vi "MS Operation Thorlabs.vi"(4 "Calib Params?":bool, 6 "OCT Z PID Gains":cluster{"Kp":dbl, "Kd":dbl, "Ki":dbl}={"Kp"=0.0003, "Kd"=0.0001, "Ki"=0.01}, 8 "error in":errorcluster, 9 "OCT Prev Posit":dbl, 11 "FPGA VI Reference In":refnum<k20>) -> (0 "error out":errorcluster, 1 "OCT Last Posit":dbl, 3 "FPGA VI Reference Out":refnum<k20>)   [LabVIEW 2016]
uses:
  <vilib>/Platform/TimedLoop/XDataNode/timing_clust.ctl
  <vilib>/Platform/TimedLoop/XDataNode/nitl_modes.ctl
  <vilib>/Platform/TimedLoop/XDataNode/wakeup.ctl
  Subsystems/Global Variables.vi
  <vilib>/Utility/error.llb/Error Cluster From Error Code.vi
  <vilib>/rvi/errors/niLvFpgaAdjustHostInterfaceError.vi
  <vilib>/platform/TimedLoop/XDataNode/XDataNode.xnode
  <vilib>/rvi/interface/nirviReadWriteControl/nirviReadWriteControl.xnode
  FPGA Bitfiles/PhantomControlPI_FPGATarget_QuadCtr2_E2412E44.lvbitx
  IRISS_FPGA_IO.vi
  <vilib>/Platform/TimedLoop/XDataNode/XDNodeRunTimeDep.lvlib
  Library/KevinLibraryAll/labview/KevLib01.lvlib
  NiFpgaLv.dll
panel:
  out "x+y 2":dbl[](array[numeric])
  out "x+y":dbl[](array[numeric])
  out "Hydration On/Off":bool
  out "vac cmd":dbl
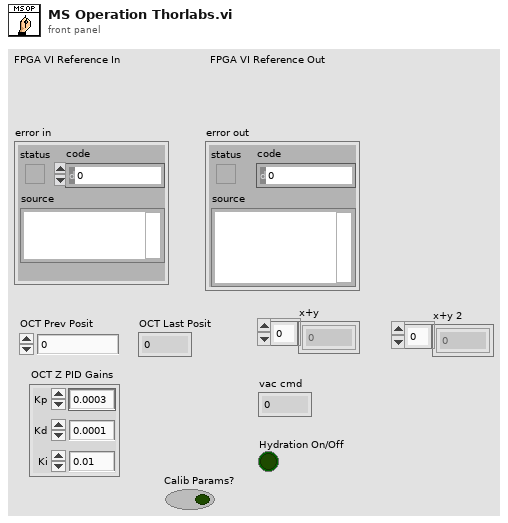
[diagram p1: front panel]
types:
  T1 = typedef "XDNodeRunTimeDep.lvlib/timing_clust.ctl" = cluster{"Expected End [f-1]":u64, "Actual End [f-1]":u64, "Finished Late? [f-1]":bool, "Expected End [i-1]":u64, "Actual End [i-1]":u64, "Finished Late? [i-1]":bool, "Expected Start [i]":u64, "Actual Start [i]":u64, "Expected Start [f]":u64, "Actual Start [f]":u64, "Source Name":string, "Structure Name":string, "Period":i64, "Deadline":i64, "Offset":i64, "Start":i64, "Priority":i32, "Timeout":i32, "Mode":T2, "Wakeup Reason":T3, "Error":errorcluster, "Source Type":string, "Secondary Source Type":string, "Global End Time":u64, "Global Start Time":u64, "Frame Duration":u64, "Iteration Duration":u64, "Assigned CPU":i32, "I/O Scan Engine Mode":u32}
  T2 = typedef "XDNodeRunTimeDep.lvlib/nitl_modes.ctl" = enum32{"No Change", "Process missed periods, maintain original phase", "Discard missed periods, maintain original phase", "Process missed periods, ignore original phase", "Discard missed periods, ignore original phase"}
  T3 = typedef "XDNodeRunTimeDep.lvlib/wakeup.ctl" = enum32{"Normal", "Aborted", "Asynchronous wakeup", "Timing source error", "Timed loop error", "Timeout"}
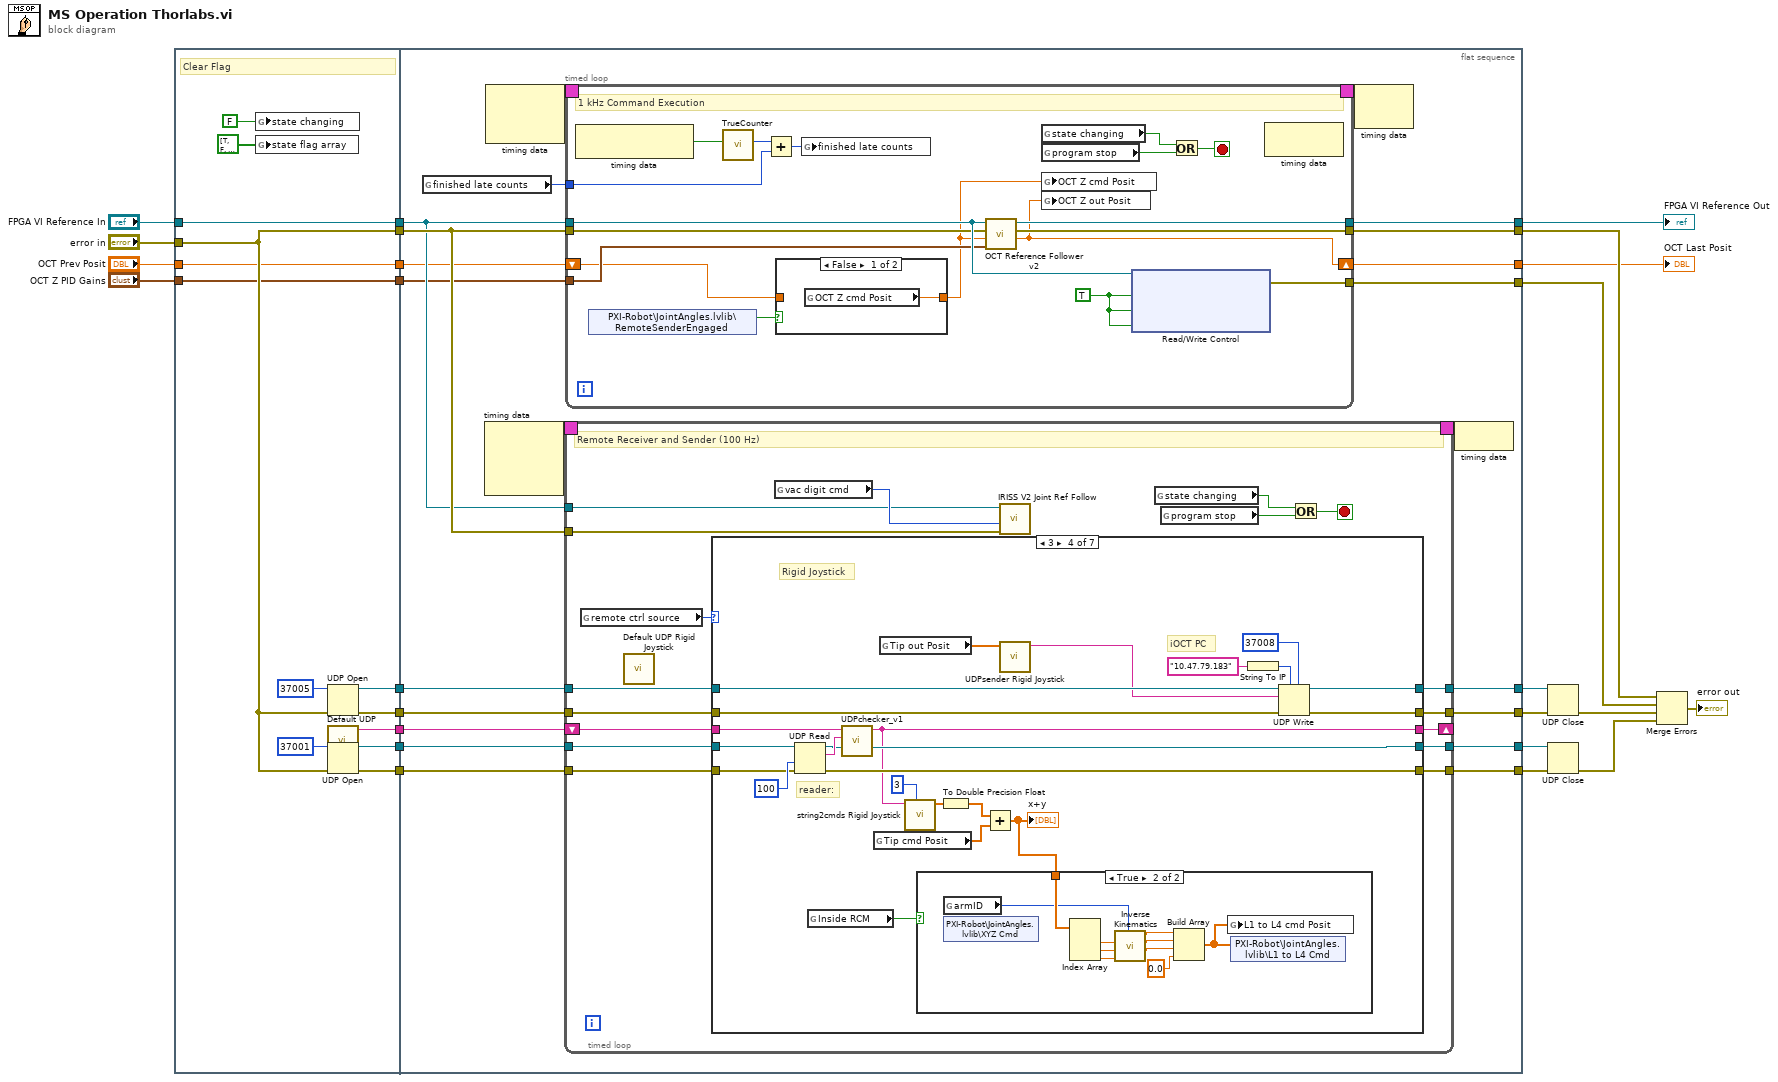
[diagram p0: block diagram]
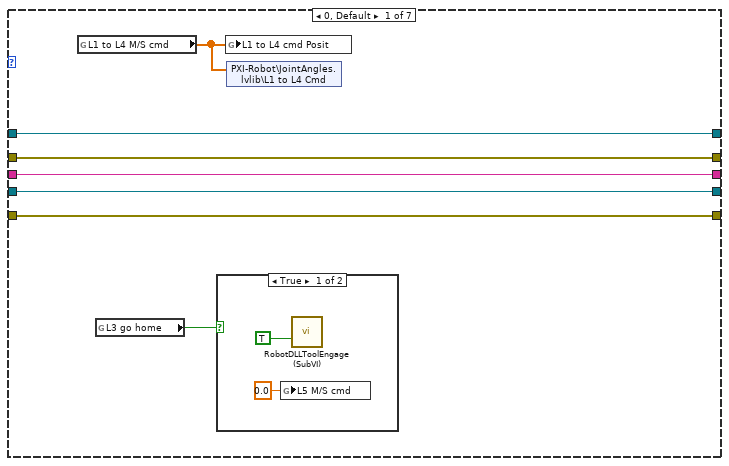
[diagram p2: hidden frame]
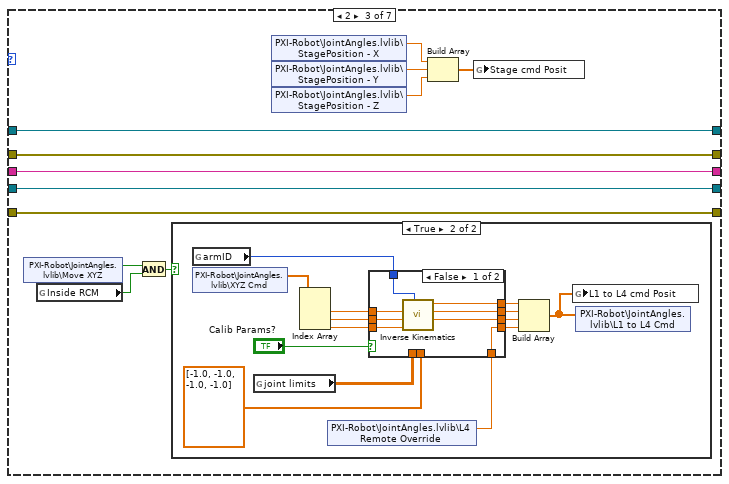
[diagram p5: hidden frame]
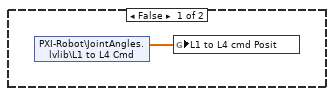
[diagram p6: hidden frame]
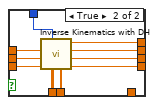
[diagram p7: hidden frame]
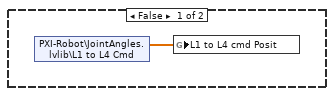
[diagram p8: hidden frame]
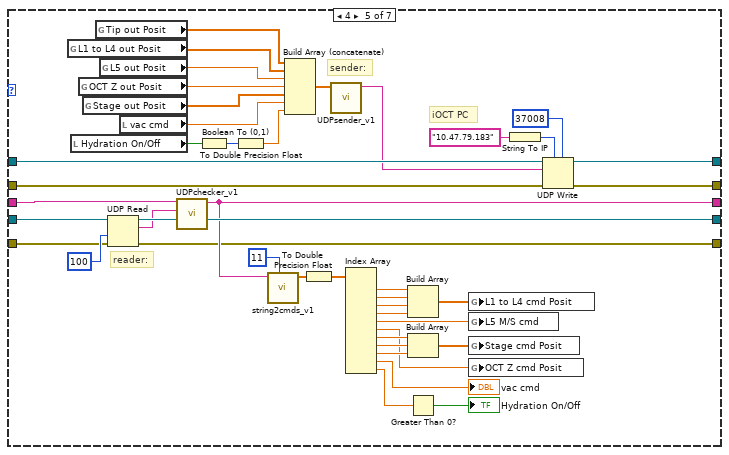
[diagram p9: hidden frame]
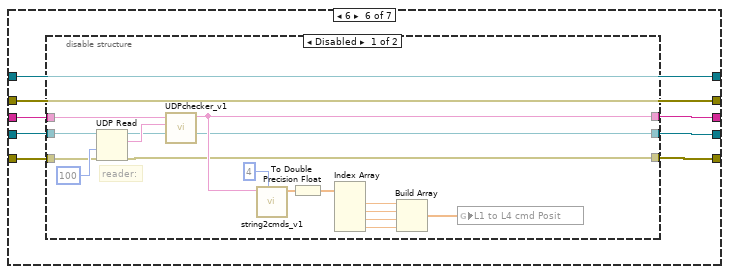
[diagram p10: hidden frame]
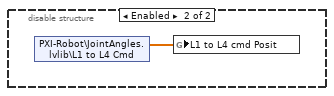
[diagram p11: hidden frame]
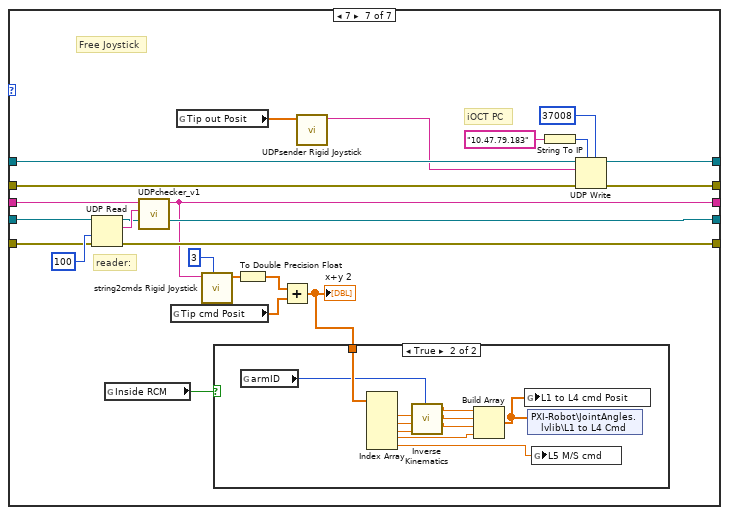
[diagram p12: hidden frame]
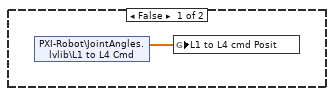
[diagram p13: hidden frame]
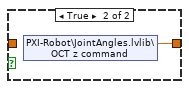
[diagram p14: hidden frame]
diagram:
  n1 = flat-sequence {
    tunnel: [w35] -> w24
    tunnel: "FPGA VI Reference In" -> [w35]
    tunnel: [w27] -> w22
    tunnel: "error in" -> [w27]
    tunnel: [w28] -> w20
    tunnel: [w32] -> w18
    tunnel: [w31] -> w17
    tunnel: [w30] -> w16
    tunnel: [w29] -> w15
    tunnel: [w26] -> w5
    tunnel: "OCT Prev Posit" -> [w26]
    tunnel: [w25] -> w3
    tunnel: "OCT Z PID Gains" -> [w25]
    tunnel: w24 -> [w41]
    tunnel: w22 -> [w42]
    tunnel: [w57] -> w6
    tunnel: [w56] -> w7
    tunnel: [w54] -> w21
    tunnel: w20 -> [w47]
    tunnel: w18 -> [w51]
    tunnel: w17 -> [w50]
    tunnel: w16 -> [w49]
    tunnel: w15 -> [w48]
    tunnel: [w46] -> w12
    tunnel: [w45] -> w11
    tunnel: [w44] -> w10
    tunnel: [w43] -> w9
    tunnel: w5 -> [w40]
    tunnel: w3 -> [w39]
    tunnel: [w38] -> w1
    frame #0 {
      # "Clear Flag"
      n2 = global write "Global Variables.vi" "state changing"(FALSE ("state changing")) -> ()
      n3 = global write "Global Variables.vi" "state flag array"(bool[] [TRUE, FALSE, FALSE, FALSE, FALSE, FALSE, FALSE, FALSE, FALSE, FALSE] ("state flag array")) -> ()
      n4 = UDP Open(8:w27, 11:u16 37005 ("port")) -> (port=w31:refnum<k16>, 0:w32:errorcluster)  [unwired: 3 in, 1 out]
      n5 = call "Default UDP.vi"() -> ("String"=w28:string)  [unwired: 11 in]
      n6 = UDP Open(8:w27, 11:u16 37001 ("port")) -> (port=w30:refnum<k16>, 0:w29:errorcluster)  [unwired: 3 in, 1 out]
    }
    frame #1 {
      n7 = global read "Global Variables.vi" "finished late counts"() -> (w55:u16)
      n8 = node-c288() -> (w53:T1)  [unwired: 3 in]
      n9 = node-c288() -> (w59:T1)  [unwired: 2 in]
      n10 = timed-loop {
        timing: w53 -> [_]
        timing-out: [_] -> w52
        tunnel: w49 -> [w76]
        tunnel: [w75] -> w44
        shift-right: [w73] -> _
        shift-left: w47 -> [w74]
        tunnel: w50 -> [w72]
        tunnel: w51 -> [w71]
        tunnel: [w70] -> w46
        tunnel: [w69] -> w45
        tunnel: w48 -> [w68]
        tunnel: [w67] -> w43
        tunnel: w41 -> [w61]
        tunnel: w42 -> [w60]
        stop <- w64 stop-if-true
        # "Remote Receiver and Sender (100 Hz)"
        n11 = global read "Global Variables.vi" "remote ctrl source"() -> (w63:u16)
        n12 = call "Default UDP Rigid Joystick.vi"() -> ()  [unwired: 11 in, 1 out]
        n13 = case shown="3" w63 {
          tunnel: w76 -> [w80 w87 w99 w156 w211 w217 w258]
          tunnel: [w80 w87 w99 w152 w210 w218 w254] -> w75
          tunnel: w74 -> [w81 w88 w100 w150 w170 w220 w252]
          tunnel: [w81 w88 w100 w149 w197 w219 w251] -> w73
          tunnel: w72 -> [w83 w90 w102 w143 w195 w213 w245]
          tunnel: w71 -> [w82 w89 w101 w141 w194 w214 w243]
          tunnel: [w83 w90 w102 w142 w190 w213 w244] -> w70
          tunnel: [w82 w89 w101 w140 w189 w214 w242] -> w69
          tunnel: w68 -> [w79 w86 w98 w155 w188 w215 w257]
          tunnel: [w79 w86 w98 w151 w187 w216 w253] -> w67
          frame 0, Default {
            n14 = global read "Global Variables.vi" "L1 to L4 M/S cmd"() -> (w77:dbl[])
            n15 = global read "Global Variables.vi" "L3 go home"() -> (w78:bool)
            n16 = case shown="True" w78 {
              frame True {
                n17 = global write "Global Variables.vi" "L5 M/S cmd"(0.0 ("L5 M/S cmd")) -> ()
                n18 = call "RobotDLLToolEngage (SubVI).vi"("Tool Fast Retraction"=TRUE ("Tool Withdraw")) -> ()  [unwired: 18 in, 1 out]
              }
              frame False {
              }
            }
            n19 = global write "Global Variables.vi" "L1 to L4 cmd Posit"(w77) -> ()
            n20 = shared-variable "PXI-Robot\\JointAngles.lvlib\\L1 to L4 Cmd"(w77) -> ()  [unwired: 1 in, 1 out]
          }
          frame 1 {
          }
          frame 2 {
            n21 = shared-variable "PXI-Robot\\JointAngles.lvlib\\Move XYZ"() -> (w96:bool)  [unwired: 1 in, 1 out]
            n22 = global read "Global Variables.vi" "Inside RCM"() -> (w95:bool)
            n23 = And(x=w96, y=w95) -> (x .and. y?=w97:bool)
            n24 = case shown="True" w97 {
              frame False {
                n25 = shared-variable "PXI-Robot\\JointAngles.lvlib\\L1 to L4 Cmd"() -> (w103:dbl[])  [unwired: 1 in, 1 out]
                n26 = global write "Global Variables.vi" "L1 to L4 cmd Posit"(w103) -> ()
              }
              frame True {
                n27 = global read "Global Variables.vi" "armID"() -> (w115:i32)
                n28 = shared-variable "PXI-Robot\\JointAngles.lvlib\\XYZ Cmd"() -> (w117:dbl[])  [unwired: 1 in, 1 out]
                n29 = global read "Global Variables.vi" "joint limits"() -> (w107:dbl[][])
                n30 = Index Array(array=w117) -> (element #1=w114:dbl, element #2=w113:dbl, element #3=w112:dbl)  [unwired: 3 in]
                n31 = shared-variable "PXI-Robot\\JointAngles.lvlib\\L4 Remote Override"() -> (w104:dbl)  [unwired: 1 in, 1 out]
                n32 = case shown="False" "Calib Params?" {
                  tunnel: w115 -> [w118 w135]
                  tunnel: w114 -> [w125 w134]
                  tunnel: w113 -> [w124 w133]
                  tunnel: w112 -> [w123 w132]
                  tunnel: [w122 w131] -> w111
                  tunnel: [w121 w130] -> w110
                  tunnel: [w120 w129] -> w109
                  tunnel: dbl[] [-1.0, -1.0, -1.0, -1.0] ("Initial guess") -> [_ w128]
                  tunnel: w107 -> [_ w127]
                  tunnel: [w119 w126] -> w106
                  tunnel: w104 -> [w119 _]
                  frame False {
                    n33 = call "Inverse Kinematics.vi"("armID"=w118, "z"=w123, "y"=w124, "x"=w125) -> ("j3"=w120:dbl, "j2"=w121:dbl, "j1"=w122:dbl)  [unwired: 4 in, 1 out]
                  }
                  frame True {
                    n34 = call "Inverse Kinematics with DH.vi"("Initial guess"=w128, "Joint Limits"=w127, "armID"=w135, "z"=w132, "y"=w133, "x"=w134) -> ("j4"=w126:dbl, "j3"=w129:dbl, "j2"=w130:dbl, "j1"=w131:dbl)  [unwired: 2 in]
                  }
                }
                n35 = Build Array(w111, w110, w109, w106) -> (w116:dbl[])
                n36 = global write "Global Variables.vi" "L1 to L4 cmd Posit"(w116) -> ()
                n37 = shared-variable "PXI-Robot\\JointAngles.lvlib\\L1 to L4 Cmd"(w116) -> ()  [unwired: 1 in, 1 out]
              }
            }
            n38 = shared-variable "PXI-Robot\\JointAngles.lvlib\\StagePosition - X"() -> (w94:dbl)  [unwired: 1 in, 1 out]
            n39 = shared-variable "PXI-Robot\\JointAngles.lvlib\\StagePosition - Y"() -> (w93:dbl)  [unwired: 1 in, 1 out]
            n40 = shared-variable "PXI-Robot\\JointAngles.lvlib\\StagePosition - Z"() -> (w92:dbl)  [unwired: 1 in, 1 out]
            n41 = Build Array(w94, w93, w92) -> (w91:dbl[])
            n42 = global write "Global Variables.vi" "Stage cmd Posit"(w91) -> ()
          }
          frame 3 {
            # "Rigid Joystick"
            # "iOCT PC"
            # "reader:"
            n43 = UDP Read(connection ID=w156, timeout ms (25000)=100, 8:w155) -> (data out=w157:string, error out=w151:errorcluster, 3:w152:refnum<k16>)  [unwired: 1 in, 2 out]
            n44 = global read "Global Variables.vi" "Inside RCM"() -> (w154:bool)
            n45 = call "UDPchecker_v1.vi"("new string"=w157, "old string"=w150) -> ("output string"=w149:string)  [unwired: 9 in]
            n46 = global read "Global Variables.vi" "Tip cmd Posit"() -> (w146:dbl[])
            n47 = global read "Global Variables.vi" "Tip out Posit"() -> (w137:dbl[])
            n48 = call "string2cmds Rigid Joystick.vi"("numCmds"=3, "input string"=w149) -> ("output cmds"=w148:dbl[])  [unwired: 9 in]
            n49 = To Double Precision Float(number=w148) -> (double precision float=w153:dbl[])
            n50 = Add(x=w153, y=w146) -> (x+y=w145:dbl[])
            "x+y" <- w145
            n51 = case shown="True" w154 {
              tunnel: w145 -> [_ w167]
              frame False {
                n52 = shared-variable "PXI-Robot\\JointAngles.lvlib\\L1 to L4 Cmd"() -> (w159:dbl[])  [unwired: 1 in, 1 out]
                n53 = global write "Global Variables.vi" "L1 to L4 cmd Posit"(w159) -> ()
              }
              frame True {
                n54 = global read "Global Variables.vi" "armID"() -> (w163:i32)
                n55 = shared-variable "PXI-Robot\\JointAngles.lvlib\\XYZ Cmd"() -> ()  [unwired: 1 in, 2 out]
                n56 = Index Array(array=w167) -> (element #1=w166:dbl, element #2=w165:dbl, element #3=w164:dbl)  [unwired: 3 in]
                n57 = call "Inverse Kinematics.vi"("armID"=w163, "z"=w164, "y"=w165, "x"=w166) -> ("j3"=w160:dbl, "j2"=w161:dbl, "j1"=w162:dbl)  [unwired: 4 in, 1 out]
                n58 = Build Array(w162, w161, w160, 0.0 ("element")) -> (w169:dbl[])
                n59 = global write "Global Variables.vi" "L1 to L4 cmd Posit"(w169) -> ()
                n60 = shared-variable "PXI-Robot\\JointAngles.lvlib\\L1 to L4 Cmd"(w169) -> ()  [unwired: 1 in, 1 out]
              }
            }
            n61 = call "UDPsender Rigid Joystick.vi"("nums2send"=w137) -> ("string2send"=w138:string)  [unwired: 10 in]
            n62 = String To IP(1:"10.47.79.183" ("name")) -> (0:w139:u32)
            n63 = UDP Write(address=w139, port or service name=u16 37008, connection ID=w143, data in=w138, 8:w141) -> (error out=w140:errorcluster, 3:w142:refnum<k16>)  [unwired: 1 in]
          }
          frame 4 {
            # "sender:"
            # "reader:"
            # "iOCT PC"
            n64 = global read "Global Variables.vi" "L1 to L4 out Posit"() -> (w180:dbl[])
            n65 = local read "Hydration On/Off"() -> (w183:bool)
            n66 = global read "Global Variables.vi" "OCT Z out Posit"() -> (w178:dbl)
            n67 = global read "Global Variables.vi" "Stage out Posit"() -> (w177:dbl[])
            n68 = global read "Global Variables.vi" "Tip out Posit"() -> (w171:dbl[])
            n69 = global read "Global Variables.vi" "L5 out Posit"() -> (w179:dbl)
            n70 = UDP Read(connection ID=w211, timeout ms (25000)=100, 8:w188) -> (data out=w196:string, error out=w187:errorcluster, 3:w210:refnum<k16>)  [unwired: 1 in, 2 out]
            n71 = local read "vac cmd"() -> (w184:dbl)
            n72 = call "UDPchecker_v1.vi"("new string"=w196, "old string"=w170) -> ("output string"=w197:string)  [unwired: 9 in]
            n73 = Boolean To (0,1)(Boolean=w183) -> (0, 1=w182:i16)
            n74 = To Double Precision Float(number=w182) -> (double precision float=w181:dbl)
            n75 = call "string2cmds_v1.vi"("numCmds"=11, "input string"=w197) -> ("output cmds"=w202:sgl[])  [unwired: 9 in]
            n76 = Build Array (concatenate)(w171, w180, w179, w178, w177, w184, w181) -> (w185:dbl[])
            n77 = To Double Precision Float(number=w202) -> (double precision float=w201:dbl[])
            n78 = call "UDPsender_v1.vi"("nums2send"=w185) -> ("string2send"=w186:string)  [unwired: 10 in]
            n79 = Index Array(array=w201) -> (element #1=w208:dbl, element #2=w207:dbl, element #3=w206:dbl, element #4=w173:dbl, element #5=w172:dbl, element #6=w175:dbl, element #7=w205:dbl, element #8=w204:dbl, element #9=w203:dbl, element #10=→"vac cmd":dbl, element #11=w199:dbl)  [unwired: 11 in]
            n80 = Build Array(w208, w207, w206, w173) -> (w174:dbl[])
            n81 = Build Array(w205, w204, w203) -> (w176:dbl[])
            n82 = Greater Than 0?(x=w199) -> (x > 0?=→"Hydration On/Off":bool)
            n83 = global write "Global Variables.vi" "L1 to L4 cmd Posit"(w174) -> ()
            n84 = global write "Global Variables.vi" "L5 M/S cmd"(w172) -> ()
            n85 = global write "Global Variables.vi" "Stage cmd Posit"(w176) -> ()
            n86 = global write "Global Variables.vi" "OCT Z cmd Posit"(w175) -> ()
            n87 = String To IP(1:"10.47.79.183" ("name")) -> (0:w192:u32)
            n88 = UDP Write(address=w192, port or service name=u16 37008, connection ID=w195, data in=w186, 8:w194) -> (error out=w189:errorcluster, 3:w190:refnum<k16>)  [unwired: 1 in]
          }
          frame 6 {
            n89 = disable-structure shown="Disabled" {
              disable-tunnel: w220 -> [w226 _]
              disable-tunnel: [w225 _] -> w219
              disable-tunnel: [w224 _] -> w218
              disable-tunnel: w217 -> [w223 _]
              disable-tunnel: [w222 _] -> w216
              disable-tunnel: w215 -> [w221 _]
              frame Disabled {
                # "reader:"
                n90 = UDP Read(connection ID=w223, timeout ms (25000)=100, 8:w221) -> (data out=w234:string, error out=w222:errorcluster, 3:w224:refnum<k16>)  [unwired: 1 in, 2 out]
                n91 = call "UDPchecker_v1.vi"("new string"=w234, "old string"=w226) -> ("output string"=w225:string)  [unwired: 9 in]
                n92 = call "string2cmds_v1.vi"("numCmds"=4, "input string"=w225) -> ("output cmds"=w232:sgl[])  [unwired: 9 in]
                n93 = To Double Precision Float(number=w232) -> (double precision float=w233:dbl[])
                n94 = Index Array(array=w233) -> (element #1=w229:dbl, element #2=w230:dbl, element #3=w231:dbl, element #4=w236:dbl)  [unwired: 4 in]
                n95 = Build Array(w229, w230, w231, w236) -> (w235:dbl[])
                n96 = global write "Global Variables.vi" "L1 to L4 cmd Posit"(w235) -> ()
              }
              frame Enabled {
                n97 = shared-variable "PXI-Robot\\JointAngles.lvlib\\L1 to L4 Cmd"() -> (w237:dbl[])  [unwired: 1 in, 1 out]
                n98 = global write "Global Variables.vi" "L1 to L4 cmd Posit"(w237) -> ()
              }
            }
          }
          frame 7 {
            # "Free Joystick"
            # "iOCT PC"
            # "reader:"
            n99 = UDP Read(connection ID=w258, timeout ms (25000)=100, 8:w257) -> (data out=w259:string, error out=w253:errorcluster, 3:w254:refnum<k16>)  [unwired: 1 in, 2 out]
            n100 = global read "Global Variables.vi" "Inside RCM"() -> (w256:bool)
            n101 = call "UDPchecker_v1.vi"("new string"=w259, "old string"=w252) -> ("output string"=w251:string)  [unwired: 9 in]
            n102 = global read "Global Variables.vi" "Tip cmd Posit"() -> (w248:dbl[])
            n103 = global read "Global Variables.vi" "Tip out Posit"() -> (w239:dbl[])
            n104 = call "string2cmds Rigid Joystick.vi"("numCmds"=3, "input string"=w251) -> ("output cmds"=w250:dbl[])  [unwired: 9 in]
            n105 = To Double Precision Float(number=w250) -> (double precision float=w255:dbl[])
            n106 = Add(x=w255, y=w248) -> (x+y=w247:dbl[])
            "x+y 2" <- w247
            n107 = case shown="True" w256 {
              tunnel: w247 -> [_ w271]
              frame False {
                n108 = shared-variable "PXI-Robot\\JointAngles.lvlib\\L1 to L4 Cmd"() -> (w261:dbl[])  [unwired: 1 in, 1 out]
                n109 = global write "Global Variables.vi" "L1 to L4 cmd Posit"(w261) -> ()
              }
              frame True {
                n110 = global read "Global Variables.vi" "armID"() -> (w267:i32)
                n111 = Index Array(array=w271) -> (element #1=w270:dbl, element #2=w269:dbl, element #3=w268:dbl, element #4=w263:dbl, element #5=w262:dbl)  [unwired: 5 in]
                n112 = call "Inverse Kinematics.vi"("armID"=w267, "z"=w268, "y"=w269, "x"=w270) -> ("j3"=w264:dbl, "j2"=w265:dbl, "j1"=w266:dbl)  [unwired: 4 in, 1 out]
                n113 = Build Array(w266, w265, w264, w263) -> (w272:dbl[])
                n114 = global write "Global Variables.vi" "L1 to L4 cmd Posit"(w272) -> ()
                n115 = shared-variable "PXI-Robot\\JointAngles.lvlib\\L1 to L4 Cmd"(w272) -> ()  [unwired: 1 in, 1 out]
                n116 = global write "Global Variables.vi" "L5 M/S cmd"(w262) -> ()
              }
            }
            n117 = call "UDPsender Rigid Joystick.vi"("nums2send"=w239) -> ("string2send"=w240:string)  [unwired: 10 in]
            n118 = String To IP(1:"10.47.79.183" ("name")) -> (0:w241:u32)
            n119 = UDP Write(address=w241, port or service name=u16 37008, connection ID=w245, data in=w240, 8:w243) -> (error out=w242:errorcluster, 3:w244:refnum<k16>)  [unwired: 1 in]
          }
        }
        n120 = global read "Global Variables.vi" "vac digit cmd"() -> (w62:i8)
        n121 = call "IRISS V2 Joint Ref Follow.vi"("error in"=w60, "Digital Cmd [0-78]"=w62, "FPGA VI Reference In"=w61) -> ()  [unwired: 5 in, 2 out]
        n122 = global read "Global Variables.vi" "state changing"() -> (w66:bool)
        n123 = global read "Global Variables.vi" "program stop"() -> (w65:bool)
        n124 = Or(x=w66, y=w65) -> (x .or. y?=w64:bool)
      }
      n125 = timed-loop {
        timing: w59 -> [_]
        timing-out: [_] -> w58
        tunnel: w41 -> [w286]
        tunnel: w42 -> [w284]
        tunnel: [w292] -> w57
        tunnel: [w285] -> w54
        tunnel: [w283] -> w56
        tunnel: w55 -> [w281]
        tunnel: w39 -> [w282]
        shift-right: [w277] -> w38
        shift-left: w40 -> [w279]
        stop <- w294 stop-if-true
        w287 = TRUE ("Conn0/DIO15 Button 4")
        # "1 kHz Command Execution"
        n126 = node-c288() -> (w290:bool)  [unwired: 1 in]
        n127 = shared-variable "PXI-Robot\\JointAngles.lvlib\\RemoteSenderEngaged"() -> (w280:bool)  [unwired: 1 in, 1 out]
        n128 = call "TrueCounter.vi"("True?"=w290) -> ("True Count"=w288:u16)  [unwired: 10 in]
        n129 = Add(x=w288, y=w281) -> (x+y=w289:u16)
        n130 = case shown="False" w280 {
          tunnel: [w295 w296] -> w278
          tunnel: w279 -> [_ _]
          frame False {
            n131 = global read "Global Variables.vi" "OCT Z cmd Posit"() -> (w295:dbl)
          }
          frame True {
            n132 = shared-variable "PXI-Robot\\JointAngles.lvlib\\OCT z command"() -> (w296:dbl)  [unwired: 1 in, 1 out]
          }
        }
        n133 = global write "Global Variables.vi" "finished late counts"(w289) -> ()
        n134 = call "OCT Reference Follower v2.vi"("OCT Z PID Gains"=w282, "OCT  Z cmd Posit [mm]"=w278, "error in"=w284, "FPGA VI Reference In"=w286) -> ("OCT  Z out Posit [mm]"=w277:dbl, "error out"=w283:errorcluster, "FPGA VI Reference Out"=w285:refnum<k20>)  [unwired: 5 in]
        n135 = global read "Global Variables.vi" "state changing"() -> (w293:bool)
        n136 = global read "Global Variables.vi" "program stop"() -> (w291:bool)
        n137 = global write "Global Variables.vi" "OCT Z cmd Posit"(w278) -> ()
        n138 = global write "Global Variables.vi" "OCT Z out Posit"(w277) -> ()
        n139 = xnode "Read/Write Control"("FPGA VI Reference In"=w286, "Conn0/DIO12 Button 1"=w287, "Conn0/DIO13 Button 2"=w287, "Conn0/DIO15 Button 4"=w287) -> ("error out"=w292:errorcluster)  [unwired: 1 in, 1 out]
        n140 = Or(x=w293, y=w291) -> (x .or. y?=w294:bool)
        n141 = node-c288() -> ()  [unwired: 1 in, 1 out]
      }
      n142 = node-c288(w58) -> ()  [unwired: 1 out]
      n143 = node-c288(w52) -> ()
    }
  }
  n144 = UDP Close(connection ID=w12, 8:w11) -> (error out=w13:errorcluster)  [unwired: 1 out]
  n145 = UDP Close(connection ID=w10, 8:w9) -> (error out=w14:errorcluster)  [unwired: 1 out]
  n146 = Merge Errors(w7, w6, w13, w14) -> (→"error out":errorcluster)
  "FPGA VI Reference Out" <- w21
  "OCT Last Posit" <- w1
